vi "PiezAlyzer.vi"() -> ()   [LabVIEW 2013]
uses:
  <vilib>/NI/STM/compatibility/stm_TCP Read Options.ctl
  <vilib>/NI/STM/TCP/Get Connection Reference (TCP).vi
  <vilib>/NI/STM/TCP/Read Message (TCP).vi
  <vilib>/NI/STM/TCP/Write Message (TCP).vi
  <vilib>/NI/STM/TCP/Read Meta Data (TCP Ref).vi
  <vilib>/NI/STM/NI STM.lvlib
  <vilib>/Analysis/NI_AALBase.lvlib
  <vilib>/Analysis/NI_AALPro.lvlib
panel:
  out "Sensitivity\n(um/V)":dbl
  in  "File Name:":string="Default"
  out "St. Dev.":dbl format="%0.2f"
  out "Mean (V)":dbl format="%0.2f"
  in  "Horizontal Pointer Slide":cluster{dbl, dbl}(slide)={0.0, 4.0} scale=-0.04010009765625..4.040802001953125 scale format="%#_2g"
  out "Loop Timing (ms)":u32
  out "Piezo Signal":dbl[](graph)
  out "XY Graph":cluster{dbl[], dbl[]}[](graph)
  in  "Record Data":bool
  in  "Tab Control":T1(tab)
  in  "Actuator sensitivity (um/V):":dbl=25.0 min=1.0 max=100.0
  in  "Experiment Name:":string="Default"
  in  "Cantilever ID:":string="Default"
  in  "Increment (um)":dbl=1.0
  in  "Down Button":bool
  in  "Up Button":bool
  out "Wave Table Duration (s):":dbl=1.0 format="%.2f"
  in  "1. Select Wave Form":T2(radio)
  in  "Amplitude (um)":dbl
  in  "Period (pts)":dbl
  in  "Duty cycle (%)":dbl
  out "Waveform Graph":dbl[](graph)
  in  "Plateau (pts)":dbl
  in  "Gain":dbl
  in  "Download":bool
  in  "Actuate!":bool
  in  "Time Interval:":i32(ring)=1000 items=["1000 ms"=1000000, "100 ms"=100000, "10 ms"=10000, "1 ms"=1000, "0.1 ms"=100]
  in  "IP Address:":string="171.64.164.81"
  in  "Connect":bool
  out "Information:":string
  in  "stop":bool
  # "Data Acquisition"
  # "TCP/IP Communication"
  # "Actuation"
  # "2. Choose its characteristics"
  # "3. Download the Wave Form to the FPGA"
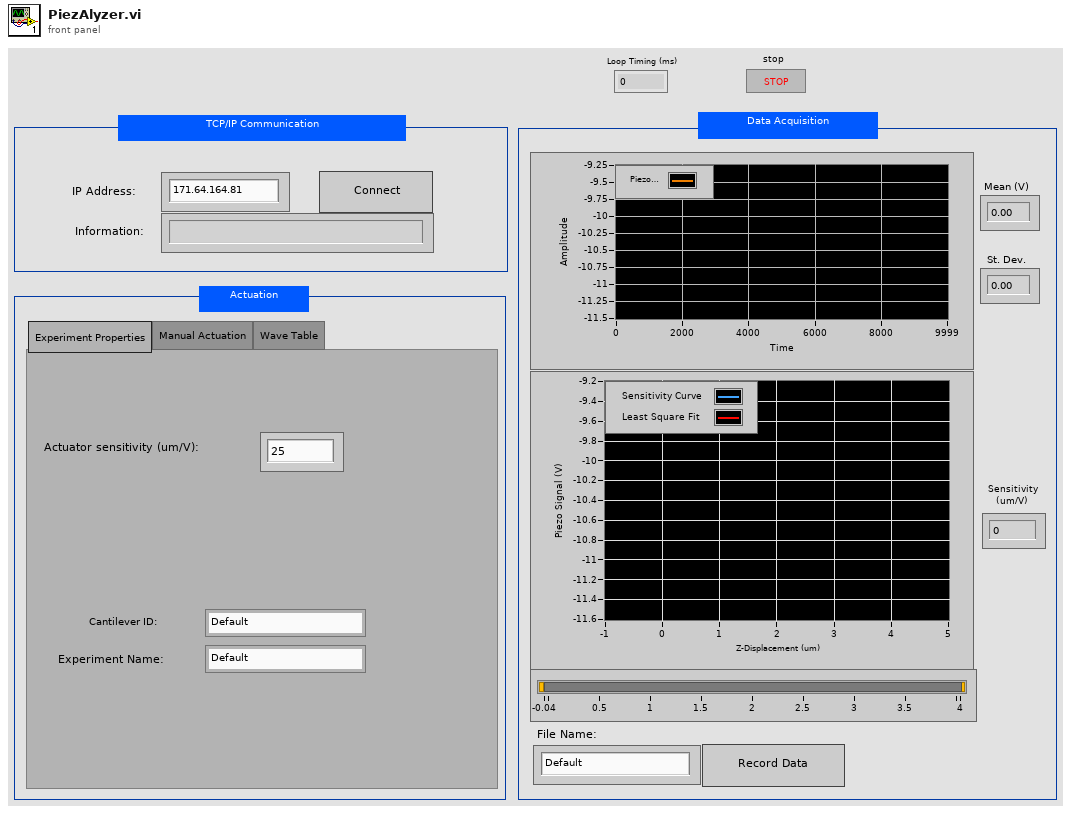
[diagram p1: front panel]
types:
  T1 = enum32{"Experiment Properties", "Manual Actuation", "Wave Table"}
  T2 = enum32{"Option 1", "Option 2", "Option 3", "Radio Selection 4", "Radio Selection 5"}
  T3 = enum16{"Stop Connexion", "Main Loop", "Try to Connect", "Idle", "Initialization"}
  T4 = typedef "stm_TCP Read Options.ctl" = cluster{"Ignore Timeout Error":bool, "timeout ms (1000)":i32}
  T5 = typedef "NI STM.lvlib/TCP Connection Info.ctl" = cluster{"connection ID":refnum<k5>, "Meta data":T6[]}
  T6 = typedef "NI STM.lvlib/MetaDataElement.ctl" = string
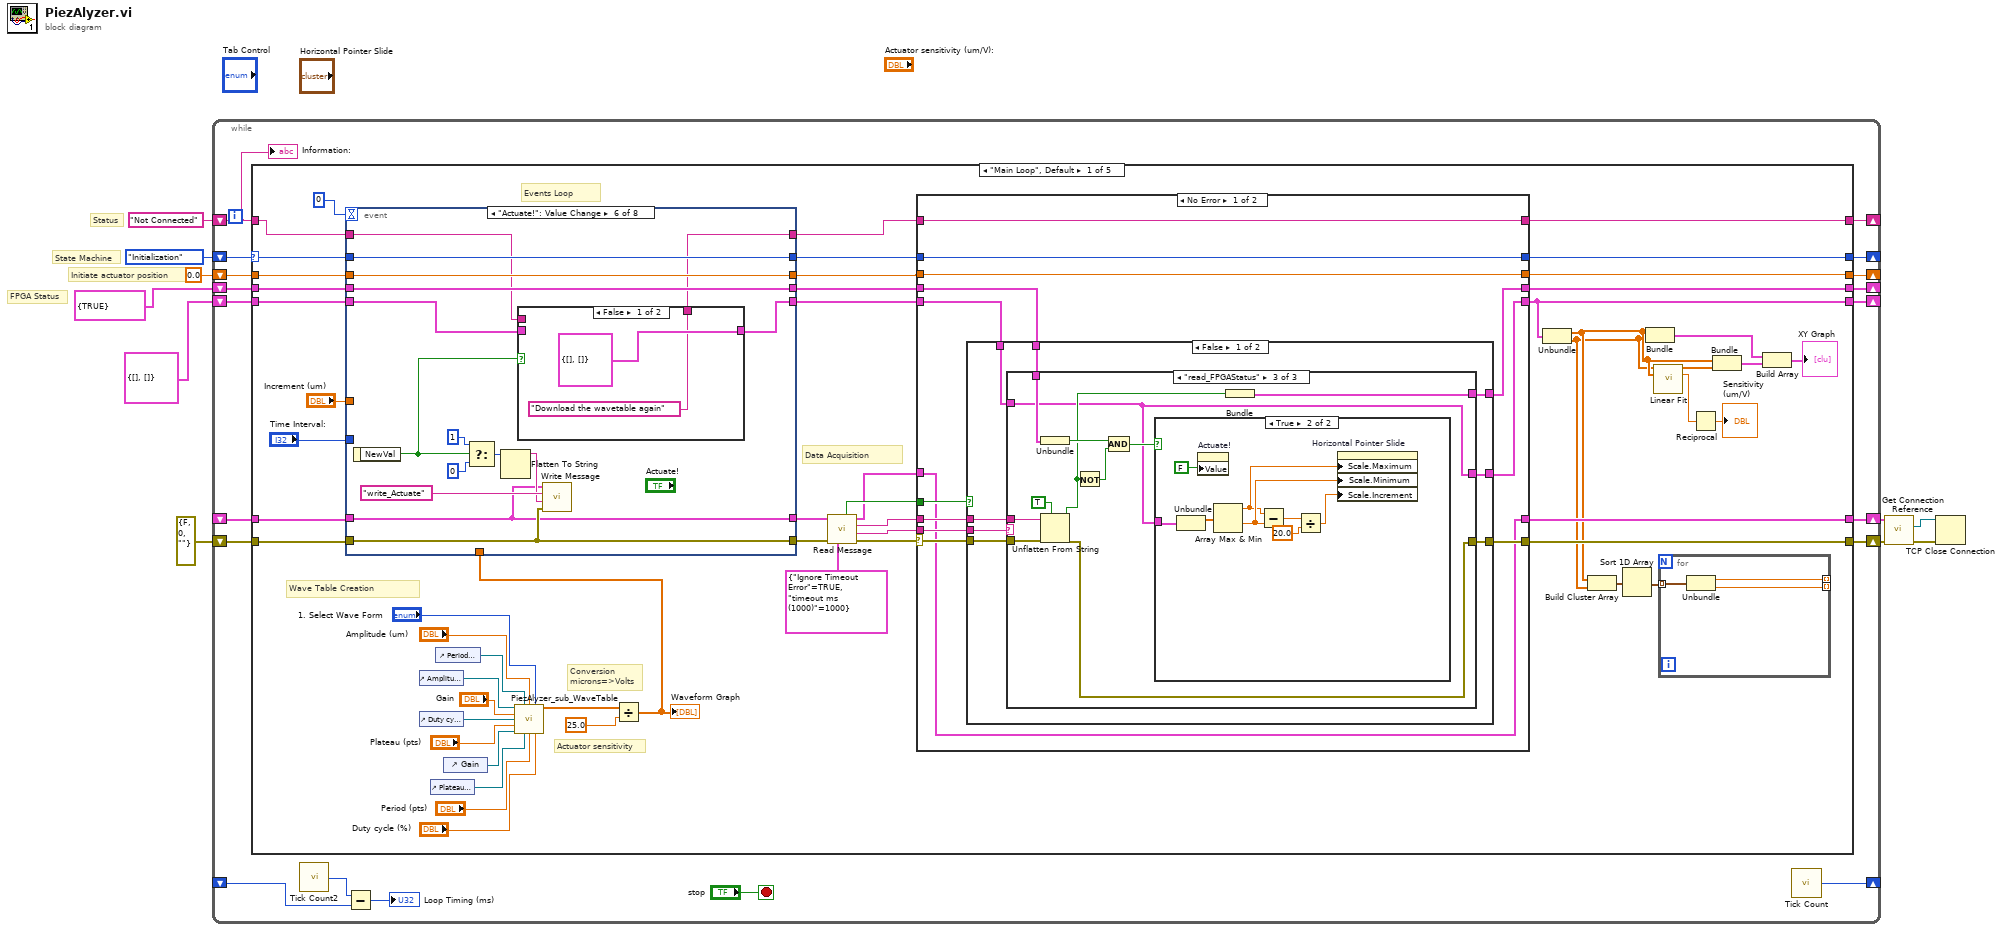
[diagram p0: block diagram]
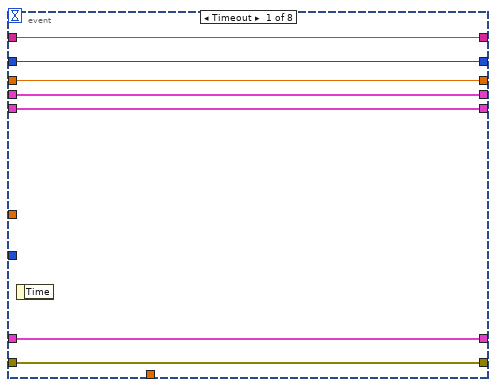
[diagram p2: hidden frame]
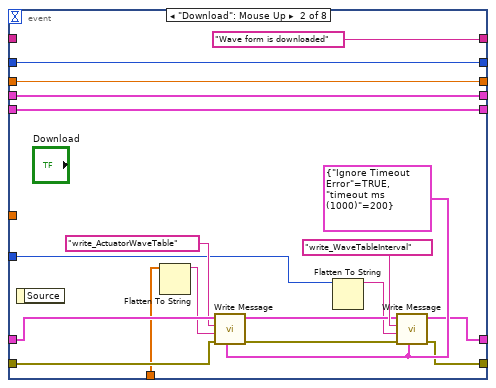
[diagram p3: hidden frame]
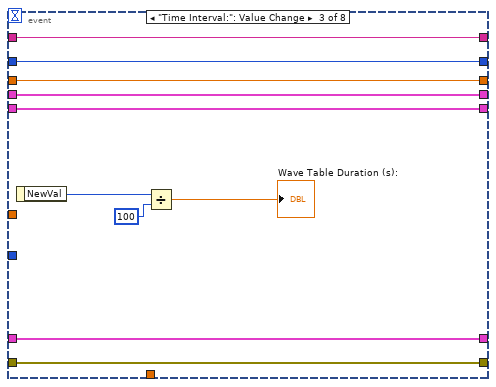
[diagram p4: hidden frame]
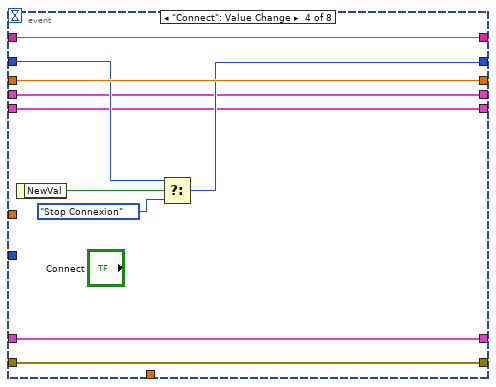
[diagram p5: hidden frame]
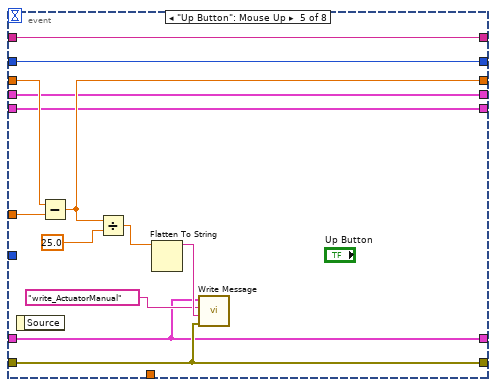
[diagram p6: hidden frame]
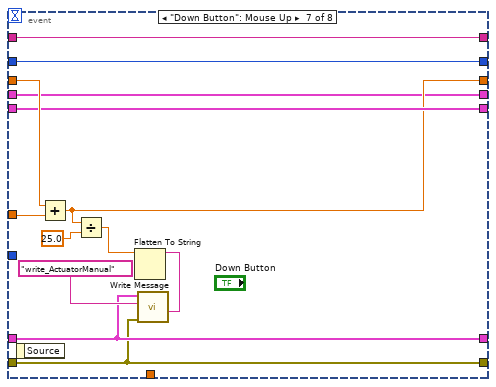
[diagram p8: hidden frame]
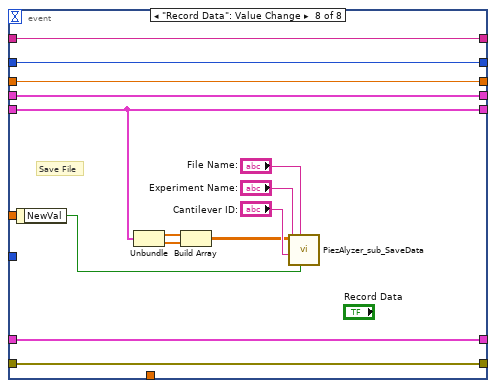
[diagram p9: hidden frame]
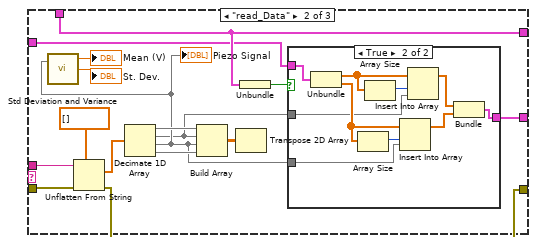
[diagram p11: hidden frame]
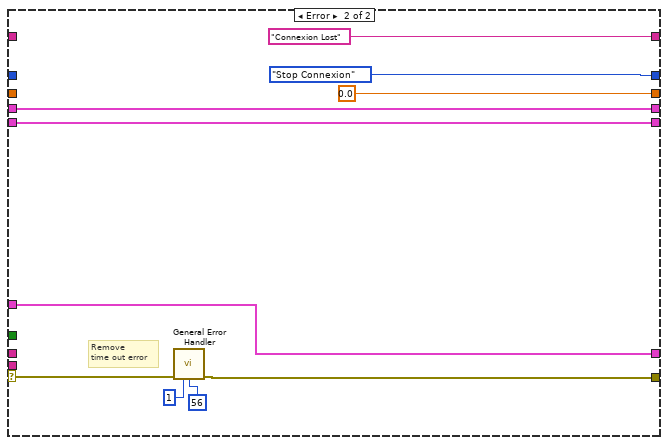
[diagram p15: hidden frame]
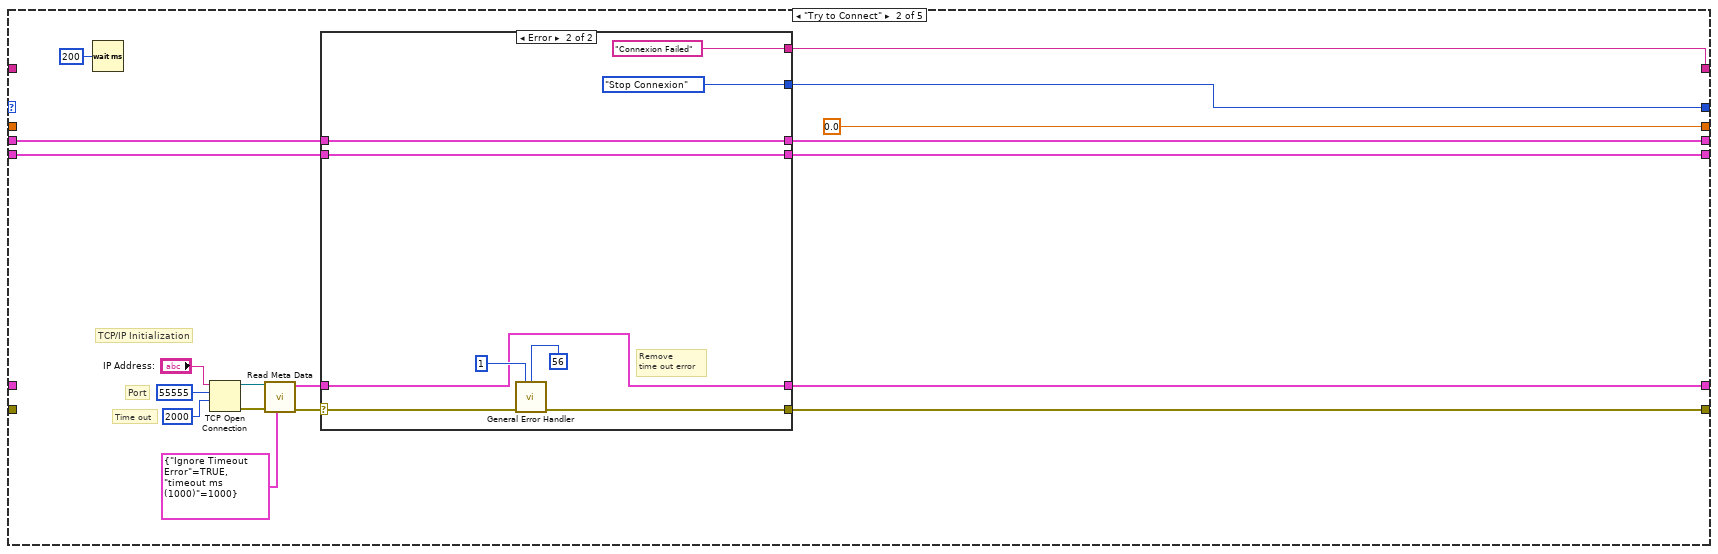
[diagram p16: hidden frame]
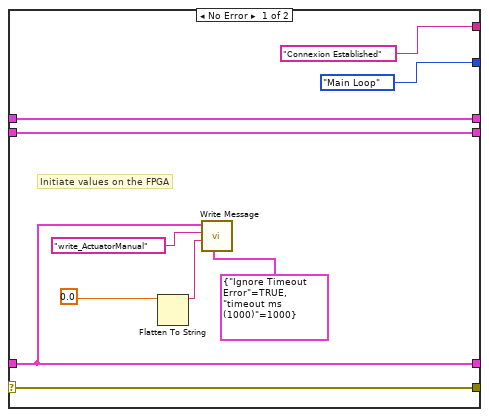
[diagram p17: hidden frame]
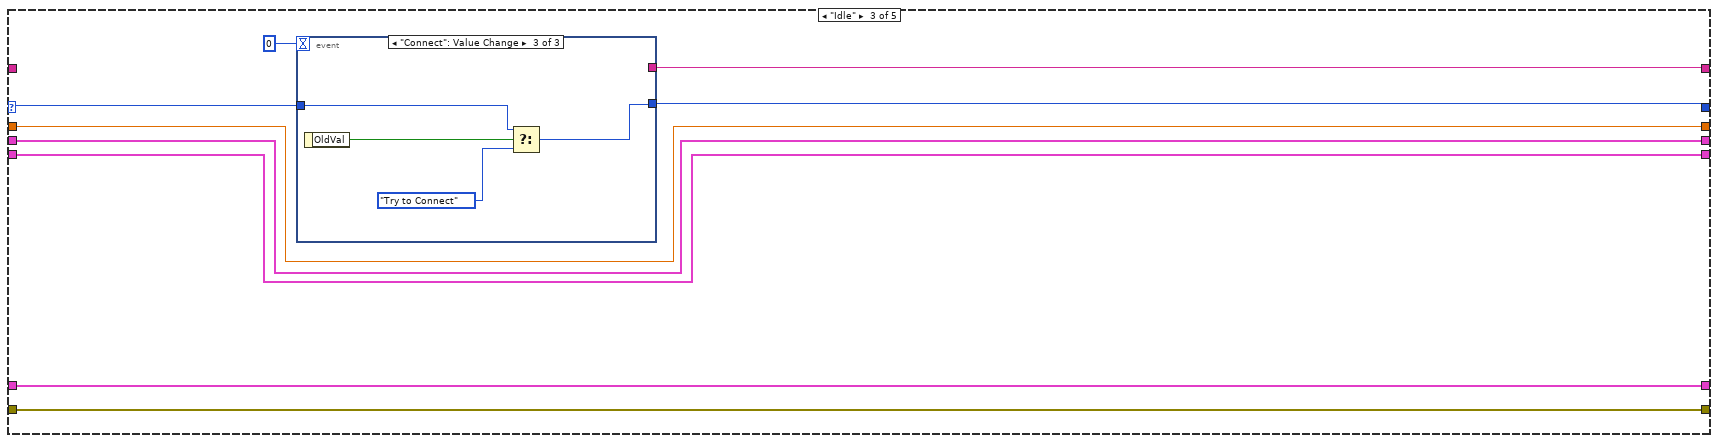
[diagram p18: hidden frame]
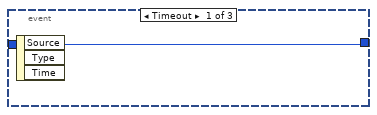
[diagram p19: hidden frame]
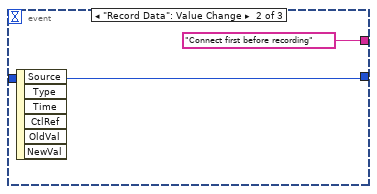
[diagram p20: hidden frame]
diagram:
  # "Status"
  # "State Machine"
  # "FPGA Status"
  # "Initiate actuator position"
  n1 = while {
    shift-right: [w22] -> _
    shift-left: T3."Initialization" -> [w25]
    shift-right: [w28] -> _
    shift-left: "Not Connected" -> [w14]
    shift-right: [w27] -> w6
    shift-left: _ -> [w24]
    shift-right: [w26] -> w5
    shift-left: errorcluster {"status"=FALSE, "code"=0, "source"=""} ("error constant") -> [w23]
    shift-right: [w20] -> _
    shift-left: 0.0 -> [w21]
    shift-right: [w17] -> _
    shift-left: _ -> [w16]
    shift-right: [w13] -> _
    shift-left: cluster{dbl[], dbl[]} {[], []} -> [w15]
    shift-right: [w12] -> _
    shift-left: cluster{bool} {TRUE} -> [w11]
    stop <- "stop" stop-if-true
    n2 = case shown="\"Main Loop\", Default" w25 {
      selector: w25 -> [w78 _ w316 _ _]
      tunnel: [w54 w285 w319 w329 "The connexion was stopped"] -> w28
      tunnel: [w51 w283 w318 w333 w336] -> w27
      tunnel: [w50 w282 w317 w332 w341] -> w26
      tunnel: w24 -> [w76 _ w318 w333 w340]
      tunnel: w23 -> [w75 _ w317 w332 w342]
      tunnel: [w53 w280 w315 T3."Idle" T3."Idle"] -> w22
      tunnel: w21 -> [w74 _ w313 w330 w337]
      tunnel: [w52 0.0 w313 w330 w337] -> w20
      tunnel: w15 -> [w57 w277 w312 w328 w335]
      tunnel: w14 -> [w45 _ _ w329 _]
      tunnel: [w36 w276 w312 w328 w335] -> w13
      tunnel: w11 -> [w49 w275 w311 w327 w334]
      tunnel: [w47 w274 w311 w327 w334] -> w12
      frame "Main Loop", Default {
        # "Data Acquisition"
        # "Events Loop"
        # "Actuator sensitivity"
        # "Wave Table Creation"
        # "Conversion \nmicrons=>Volts"
        n3 = control-ref of="Amplitude (um)"() -> (w69:refnum<vi>)
        n4 = control-ref of="Duty cycle (%)"() -> (w71:refnum<vi>)
        n5 = control-ref of="Plateau (pts)"() -> (w73:refnum<vi>)
        n6 = control-ref of="Period (pts)"() -> (w70:refnum<vi>)
        n7 = control-ref of="Gain"() -> (w72:refnum<vi>)
        n8 = call "PiezAlyzer_sub_WaveTable.vi"("Digital in"=w69, "reference in"=w70, "Amplitude (um)"="Amplitude (um)", "1. Select Wave Form"="1. Select Wave Form", "Gain"="Gain", "reference 3"=w71, "Plateau (ms)"="Plateau (pts)", "reference 4"=w72, "reference 5"=w73, "Period (ms)"="Period (pts)", "Duty cycle (%)"="Duty cycle (%)") -> ("Array"=w67:dbl[])  [unwired: 4 in]
        n9 = Divide(x=w67, y=25.0) -> (x/y=w56:dbl[])
        "Waveform Graph" <- w56
        n10 = event shown="[5] \"Actuate!\": Value Change" {
          selector: _ -> [_ _ _ _ _ _ _ _]
          dyn-events: _ -> [_ _ _ _ _ _ _ _]
          timeout: 0 -> [_ _ _ _ _ _ _ _]
          tunnel: [w92 w110 w120 w128 w138 w153 w171 w190] -> w59
          tunnel: w76 -> [w91 w104 w116 w126 w134 w148 w167 w188]
          tunnel: "Increment (um)" -> [_ _ _ _ w137 _ w173 _]
          tunnel: w74 -> [w93 w111 w119 w130 w141 w159 w170 w189]
          tunnel: [w93 w111 w119 w130 w139 w159 w168 w189] -> w58
          tunnel: w75 -> [w90 w105 w115 w125 w135 w149 w166 w187]
          tunnel: [w90 w96 w115 w125 w135 w149 w166 w187] -> w60
          tunnel: [w91 w95 w116 w126 w134 w148 w167 w188] -> w43
          tunnel: w78 -> [w92 w110 w120 w127 w138 w153 w171 w190]
          tunnel: w56 -> [_ w103 _ _ _ _ _ _]
          tunnel: w57 -> [w89 w108 w117 w124 w136 w150 w169 w182]
          tunnel: [w89 w108 w117 w124 w136 w152 w169 w182] -> w31
          tunnel: w49 -> [w88 w109 w118 w123 w133 w147 w165 w178]
          tunnel: [w88 w109 w118 w123 w133 w147 w165 w178] -> w48
          tunnel: w45 -> [w87 _ w121 w122 w132 w145 w164 w177]
          tunnel: [w87 "Wave form is downloaded" w121 w122 w132 w146 w164 w177] -> w44
          tunnel: "Time Interval:" -> [_ w94 _ _ _ _ _ _]
          event Timeout {
            n11 = event-data() -> ()  [unwired: 1 in, 1 out]
          }
          event "Download": Mouse Up {
            w97 = T4 {"Ignore Timeout Error"=TRUE, "timeout ms (1000)"=200} ("Options")
            n12 = event-data() -> ()  [unwired: 1 in, 1 out]
            n13 = Flatten To String(anything=w103) -> (data string=w102:string)  [unwired: 3 in, 2 out]
            n14 = call-poly <vilib>:"Write Message.vi"("Options"=w97, "error in (no error)"=w105, "Data"=w102, "Name"="write_ActuatorWaveTable", "Connection Info"=w104) -> ("error out"=w99:errorcluster, "Connection Info Out"=w100:T5)  [unwired: 5 in]
            n15 = Flatten To String(anything=w94) -> (data string=w98:string)  [unwired: 3 in, 2 out]
            n16 = call-poly <vilib>:"Write Message.vi"("Options"=w97, "error in (no error)"=w99, "Data"=w98, "Name"="write_WaveTableInterval", "Connection Info"=w100) -> ("error out"=w96:errorcluster, "Connection Info Out"=w95:T5)  [unwired: 5 in]
          }
          event "Time Interval:": Value Change {
            n17 = event-data() -> ("NewVal"=w114:i32)  [unwired: 1 in]
            n18 = Divide(x=w114, y=100) -> (x/y=→"Wave Table Duration (s):":dbl)
          }
          event "Connect": Value Change {
            n19 = event-data() -> ("NewVal"=w129:bool)  [unwired: 1 in]
            n20 = Select(t=w127, s=w129, f=T3."Stop Connexion") -> (s? t:f=w128:T3)
          }
          event "Up Button": Mouse Up {
            n21 = event-data() -> ()  [unwired: 1 in, 1 out]
            n22 = Subtract(x=w141, y=w137) -> (x-y=w139:dbl)
            n23 = Divide(x=w139, y=25.0) -> (x/y=w140:dbl)
            n24 = Flatten To String(anything=w140) -> (data string=w143:string)  [unwired: 3 in, 2 out]
            n25 = call-poly <vilib>:"Write Message.vi"("error in (no error)"=w135, "Data"=w143, "Name"="write_ActuatorManual", "Connection Info"=w134) -> ()  [unwired: 6 in, 2 out]
          }
          event "Actuate!": Value Change {
            n26 = event-data() -> ("NewVal"=w151:bool)  [unwired: 1 in]
            n27 = Select(t=1, s=w151, f=0) -> (s? t:f=w156:i32)
            n28 = Flatten To String(anything=w156) -> (data string=w157:string)  [unwired: 3 in, 2 out]
            n29 = case shown="False" w151 {
              tunnel: [cluster{dbl[], dbl[]} {[], []} w163] -> w152
              tunnel: w150 -> [_ w163]
              tunnel: ["Download the wavetable again" w162] -> w146
              tunnel: w145 -> [_ w162]
              frame False {
              }
              frame True {
              }
            }
            n30 = call-poly <vilib>:"Write Message.vi"("error in (no error)"=w149, "Data"=w157, "Name"="write_Actuate", "Connection Info"=w148) -> ()  [unwired: 6 in, 2 out]
          }
          event "Down Button": Mouse Up {
            n31 = event-data() -> ()  [unwired: 1 in, 1 out]
            n32 = Add(x=w170, y=w173) -> (x+y=w168:dbl)
            n33 = Divide(x=w168, y=25.0) -> (x/y=w172:dbl)
            n34 = Flatten To String(anything=w172) -> (data string=w175:string)  [unwired: 3 in, 2 out]
            n35 = call-poly <vilib>:"Write Message.vi"("error in (no error)"=w166, "Data"=w175, "Name"="write_ActuatorManual", "Connection Info"=w167) -> ()  [unwired: 6 in, 2 out]
          }
          event "Record Data": Value Change {
            # "Save File"
            n36 = event-data() -> ("NewVal"=w183:bool)  [unwired: 1 in]
            n37 = Unbundle(w182) -> (w181:dbl[], w180:dbl[])
            n38 = Build Array(w181, w180) -> (w179:dbl[][])
            n39 = call "PiezAlyzer_sub_SaveData.vi"("Boolean"=w183, "File Name:"="File Name:", "Cantilever ID:"="Cantilever ID:", "Experiment Name:"="Experiment Name:", "Array"=w179) -> ()  [unwired: 7 in]
          }
        }
        n40 = call-poly <vilib>:"Read Message.vi"("Options"=T4 {"Ignore Timeout Error"=TRUE, "timeout ms (1000)"=1000}, "error in"=w60, "Connection Info"=w43) -> ("error out"=w82:errorcluster, "Name"=w80:T6, "data string"=w81:string, "Connection Info Out"=w79:T5, "Timed Out?"=w83:bool)  [unwired: 3 in, 1 out]
        n41 = case shown="No Error" w82 {
          selector: w82 -> [w199 w266]
          tunnel: w80 -> [w200 _]
          tunnel: w81 -> [w201 _]
          tunnel: w83 -> [w203 _]
          tunnel: [w196 w265] -> w50
          tunnel: [w195 w267] -> w51
          tunnel: w44 -> [w202 _]
          tunnel: [w202 "Connexion Lost"] -> w54
          tunnel: [w198 T3."Stop Connexion"] -> w53
          tunnel: [w197 0.0] -> w52
          tunnel: w79 -> [w195 w267]
          tunnel: [w191 w268] -> w36
          tunnel: w59 -> [w198 _]
          tunnel: w58 -> [w197 _]
          tunnel: w31 -> [w192 w268]
          tunnel: w48 -> [w193 w264]
          tunnel: [w194 w264] -> w47
          frame No Error {
            n42 = case shown="False" w203 {
              tunnel: w200 -> [w209 _]
              tunnel: w201 -> [w211 _]
              tunnel: w199 -> [w210 w263]
              tunnel: [w208 w263] -> w196
              tunnel: [w207 w262] -> w194
              tunnel: w193 -> [w206 w262]
              tunnel: w192 -> [w205 w261]
              tunnel: [w204 w261] -> w191
              frame False {
                n43 = case shown="\"read_FPGAStatus\"" w209 {
                  tunnel: w211 -> [_ w225 w252]
                  tunnel: w210 -> [w214 w224 w251]
                  tunnel: [w214 w221 w244] -> w208
                  tunnel: [w213 w220 w249] -> w207
                  tunnel: w206 -> [w213 w220 w248]
                  tunnel: w205 -> [w212 w218 w242]
                  tunnel: [w212 w215 w242] -> w204
                  frame Default {
                  }
                  frame "read_Data" {
                    n44 = Unflatten From String(type=dbl[] [], binary string=w225, error in (no error)=w224) -> (value=w229:dbl[], error out=w221:errorcluster)  [unwired: 3 out]
                    n45 = Decimate 1D Array(w229) -> (w226:dbl[], w216:dbl[], w217:dbl[], w227:dbl[])
                    "Piezo Signal" <- w217
                    n46 = call <vilib>:"Std Deviation and Variance.vi"("X"=w217) -> ("mean"=→"Mean (V)":dbl, "standard deviation"=→"St. Dev.":dbl)  [unwired: 1 in, 1 out]
                    n47 = Build Array(w226, w216, w217, w227) -> (w228:dbl[][])
                    n48 = Transpose 2D Array(2D array=w228) -> ()  [unwired: 1 out]
                    n49 = Unbundle(w220) -> (w219:bool)
                    n50 = case shown="True" w219 {
                      tunnel: w218 -> [w231 w239]
                      tunnel: w217 -> [_ w236]
                      tunnel: w216 -> [_ w235]
                      tunnel: [w231 w232] -> w215
                      frame False {
                      }
                      frame True {
                        n51 = Unbundle(w239) -> (w241:dbl[], w237:dbl[])
                        n52 = Array Size(array=w237) -> (size(s)=w238:i32)
                        n53 = Array Size(array=w241) -> (size(s)=w240:i32)
                        n54 = Insert Into Array(array=w237, index=w238, new element=w236) -> (w234:dbl[])
                        n55 = Insert Into Array(array=w241, index=w240, new element=w235) -> (w233:dbl[])
                        n56 = Bundle(w233, w234) -> (w232:cluster{dbl[], dbl[]})  [unwired: 1 in]
                      }
                    }
                  }
                  frame "read_FPGAStatus" {
                    n57 = Unbundle(w248) -> (w247:bool)
                    n58 = Unflatten From String(type=TRUE, binary string=w252, error in (no error)=w251) -> (value=w243:bool, error out=w244:errorcluster)  [unwired: 3 out]
                    n59 = Not(x=w243) -> (.not. x?=w246:bool)
                    n60 = And(x=w247, y=w246) -> (x .and. y?=w245:bool)
                    n61 = case shown="True" w245 {
                      tunnel: w242 -> [_ w253]
                      frame False {
                      }
                      frame True {
                        n62 = Unbundle(w253) -> (w254:dbl[])  [unwired: 1 out]
                        n63 = property on="Actuate!" class="Bool (strict)"("Value"=FALSE) -> ()  [unwired: 2 in, 2 out]
                        n64 = Array Max & Min(array=w254) -> (max value=w258:dbl, min value=w259:dbl)  [unwired: 2 out]
                        n65 = Subtract(x=w258, y=w259) -> (x-y=w257:dbl)
                        n66 = Divide(x=w257, y=20.0) -> (x/y=w255:dbl)
                        n67 = property on="Horizontal Pointer Slide" class="Slide (strict)"("Scale.Maximum"=w258, "Scale.Minimum"=w259, "Scale.Increment"=w255) -> ()  [unwired: 2 in, 2 out]
                      }
                    }
                    n68 = Bundle(w243) -> (w249:cluster{bool})  [unwired: 1 in]
                  }
                }
              }
              frame True {
              }
            }
          }
          frame Error {
            # "Remove \ntime out error"
            n69 = call <vilib>:"General Error Handler.vi"("error in (no error)"=w266, "[exception action] (none:0)"=1, "[exception code]"=56) -> ("error out"=w265:errorcluster)  [unwired: 8 in, 4 out]
          }
        }
        n70 = Unbundle(w36) -> (w35:dbl[], w34:dbl[])
        n71 = Build Cluster Array(w35, w34) -> (w33:cluster{dbl, dbl}[])
        n72 = Sort 1D Array(array=w33) -> (sorted array=w32:cluster{dbl, dbl}[])
        n73 = Bundle(w35, w34) -> (w38:cluster{dbl[], dbl[]})  [unwired: 1 in]
        n74 = call <vilib>:"Linear Fit.vi"("Y"=w34, "X"=w35) -> ("Best Linear Fit"=w39:dbl[], "slope"=w42:dbl)  [unwired: 9 in, 3 out]
        n75 = for {
          tunnel: w32 -> [w86] mode=indexing
          tunnel: [w85] -> _ mode=indexing
          tunnel: [w84] -> _ mode=indexing
          n76 = Unbundle(w86) -> (w85:dbl, w84:dbl)
        }
        n77 = Reciprocal(x=w42) -> (1/x=→"Sensitivity\n(um/V)":dbl)
        n78 = Bundle(w35, "Best Linear Fit"=w39) -> (w40:cluster{dbl[], "Best Linear Fit":dbl[]})  [unwired: 1 in]
        n79 = Build Array(w38, w40) -> (→"XY Graph":cluster{dbl[], "Best Linear Fit":dbl[]}[])
      }
      frame "Try to Connect" {
        # "Time out"
        # "Port"
        # "TCP/IP Initialization"
        n80 = Wait (ms)(milliseconds to wait=200) -> ()  [unwired: 1 out]
        n81 = TCP Open Connection(address="IP Address:", remote port or service name=u16 55555 ("remote port"), timeout ms (60000)=u16 2000 ("remote port")) -> (connection ID=w290:refnum<k5>, error out=w291:errorcluster)  [unwired: 1 in, 1 out]
        n82 = call-poly <vilib>:"Read Meta Data.vi"("Options"=T4 {"Ignore Timeout Error"=TRUE, "timeout ms (1000)"=1000}, "error in"=w291, "connection ID"=w290) -> ("error out"=w286:errorcluster, "Connection Info Out"=w284:T5)  [unwired: 6 in, 1 out]
        n83 = case shown="Error" w286 {
          selector: w286 -> [w300 w310]
          tunnel: ["Connexion Established" "Connexion Failed"] -> w285
          tunnel: [T3."Main Loop" T3."Stop Connexion"] -> w280
          tunnel: [w296 w305] -> w283
          tunnel: w284 -> [w296 w305]
          tunnel: [w300 w304] -> w282
          tunnel: [w293 w303] -> w276
          tunnel: w277 -> [w293 w303]
          tunnel: w275 -> [w292 w302]
          tunnel: [w292 w302] -> w274
          frame No Error {
            # "Initiate values on the FPGA"
            n84 = Flatten To String(anything=0.0) -> (data string=w298:string)  [unwired: 3 in, 2 out]
            n85 = call-poly <vilib>:"Write Message.vi"("Options"=T4 {"Ignore Timeout Error"=TRUE, "timeout ms (1000)"=1000}, "Data"=w298, "Name"="write_ActuatorManual", "Connection Info"=w296) -> ()  [unwired: 6 in, 2 out]
          }
          frame Error {
            # "Remove \ntime out error"
            n86 = call <vilib>:"General Error Handler.vi"("error in (no error)"=w310, "[exception action] (none:0)"=1, "[exception code]"=56) -> ("error out"=w304:errorcluster)  [unwired: 8 in, 4 out]
          }
        }
      }
      frame "Idle" {
        n87 = event shown="[2] \"Connect\": Value Change" {
          selector: _ -> [_ _ _]
          dyn-events: _ -> [_ _ _]
          timeout: 0 -> [_ _ _]
          tunnel: [_ "Connect first before recording" _] -> w319
          tunnel: w316 -> [w320 w321 w325]
          tunnel: [w320 w321 w324] -> w315
          event Timeout {
            n88 = event-data() -> ()  [unwired: 1 in, 3 out]
          }
          event "Record Data": Value Change {
            n89 = event-data() -> ()  [unwired: 1 in, 6 out]
          }
          event "Connect": Value Change {
            n90 = event-data() -> ("OldVal"=w323:bool)  [unwired: 1 in]
            n91 = Select(t=w325, s=w323, f=T3."Try to Connect") -> (s? t:f=w324:T3)
          }
        }
      }
      frame "Initialization" {
      }
      frame "Stop Connexion" {
        # "Close the TCP\nconnexion"
        n92 = call-poly <vilib>:"Get Connection Reference.vi"("error in"=w342, "Connection Info"=w340) -> ("error out"=w343:errorcluster, "connection ID out"=w344:refnum<k5>, "Connection Info Out"=w336:T5)  [unwired: 7 in]
        n93 = TCP Close Connection(connection ID=w344, error in (no error)=w343) -> (error out=w341:errorcluster)  [unwired: 2 out]
      }
    }
    n94 = call "Tick Count2"() -> ("Tick Count(mSec)"=w19:u32)
    n95 = Subtract(x=w19, y=w16) -> (x-y=→"Loop Timing (ms)":u32)
    n96 = call "Tick Count"() -> ("Tick Count(mSec)"=w17:u32)
    "Information:" <- w14
  }
  n97 = call-poly <vilib>:"Get Connection Reference.vi"("error in"=w5, "Connection Info"=w6) -> ("error out"=w10:errorcluster, "connection ID out"=w9:refnum<k5>)  [unwired: 7 in, 1 out]
  n98 = TCP Close Connection(connection ID=w9, error in (no error)=w10) -> ()  [unwired: 3 out]
